vi "_UTIL_Run_TestVector File.vi"() -> ()   [LabVIEW 2024]
uses:
  Control Definitions/Def FullCfg.ctl
  Control Definitions/Def BenchCfg.ctl
  Control Definitions/Def PumpCtlRefs.ctl
  Control Definitions/Def Bench Status.ctl
  Control Definitions/Ded Spec RNG.ctl
  Control Definitions/Ded LUT_Status.ctl
  Control Definitions/Def Results2.ctl
panel:
  out "Time":dbl
  out "Point #":i32
  out "File Name":string
  out "Root path":path
  out "Results out":T1=[[{"Fill"=0.0, "Drain"=7.612782182151588, "Status"=5, "Resistor"=100.2}, {"Fill"=3.699999999999991, "Drain"=7.368700152811735, "Status"=9, "Resistor"=100.4}], [{"Fill"=7.519750916870415, "Drain"=7.144624847188264, "Status"=5, "Resistor"=199.3}, {"Fill"=7.323685024449877, "Drain"=6.908545507334963, "Status"=5, "Resistor"=199.4}], [{"Fill"=7.101610391198044, "Drain"=6.69747457212714, "Status"=5, "Resistor"=298.5}, {"Fill"=6.859529034229828, "Drain"=6.46039489608802, "Status"=5, "Resistor"=298.4}], [{"Fill"=6.616447341075794, "Drain"=6.23331858190709, "Status"=5, "Resistor"=397.6}, {"Fill"=6.4163801039119805, "Drain"=6.007242603911981, "Status"=5, "Resistor"=397.6}], [{"Fill"=6.176299419315403, "Drain"=5.775164608801956, "Status"=5, "Resistor"=497.4}, {"Fill"=5.938219407090465, "Drain"=5.544086949877751, "Status"=5, "Resistor"=497.2}], [{"Fill"=5.733150488997555, "Drain"=5.331015342298288, "Status"=5, "Resistor"=597.7}, {"Fill"=5.478064761613692, "Drain"=5.0889339853300735, "Status"=5, "Resistor"=597.0}], [{"Fill"=5.25498979217604, "Drain"=4.853854981662591, "Status"=5, "Resistor"=697.7}, {"Fill"=5.02791347799511, "Drain"=4.634781356968215, "Status"=5, "Resistor"=697.0}], [{"Fill"=4.795835482885085, "Drain"=4.415707732273838, "Status"=5, "Resistor"=797.9}, {"Fill"=4.572760513447433, "Drain"=0.0, "Status"=5, "Resistor"=797.2}], [{"Fill"=4.368691931540343, "Drain"=3.9545527506112466, "Status"=5, "Resistor"=897.6}, {"Fill"=4.125610238386308, "Drain"=4.172626039119804, "Status"=10, "Resistor"=856.6}], [{"Fill"=3.90853728606357, "Drain"=0.0, "Status"=5, "Resistor"=998.1}, {"Fill"=3.68246130806846, "Drain"=3.7114710574572127, "Status"=10, "Resistor"=897.1}], [{"Fill"=3.45638533007335, "Drain"=3.389362805623472, "Status"=10, "Resistor"=998.3}, {"Fill"=3.200299266503668, "Drain"=3.010235391198044, "Status"=10, "Resistor"=997.4}]] {"Resistor" format="%.1f"; "Drain" format="%.3f"; "Fill" format="%.3f"}
  in  "aSpec Out":T2[](array[typedef])
  out "Fill!Drain":bool=TRUE
  in  "Full Config":T4={"Bench Config"={"Name"="OLR001", {"Step Levels"=0.05, "Tolerance"=0.01, "Sample Rate"=0.05, "Resistor"=100.0, "M Level Cal"=1.0, "[B Level Cal"=0.0, "Max Fill Rate"=0.025, "Empty Inches"=8.6, "Full Inches"=2.0}}, "Test Value Table "=[[98.0, 102.0, 7.91, 8.01, 7.55, 7.65, 98.0, 102.0, 7.685, 7.785, 7.325, 7.425], [197.0, 203.0, 7.46, 7.56, 7.1, 7.2, 197.0, 203.0, 7.235, 7.335, 6.875, 6.975], [296.0, 304.0, 7.01, 7.11, 6.65, 6.75, 296.0, 304.0, 6.785, 6.885, 6.425, 6.525], [395.0, 405.0, 6.56, 6.66, 6.2, 6.3, 395.0, 405.0, 6.335, 6.435, 5.975, 6.075], [494.0, 506.0, 6.11, 6.21, 5.75, 5.85, 494.0, 506.0, 5.885, 5.985, 5.525, 5.625], [593.0, 607.0, 5.66, 5.76, 5.3, 5.4, 593.0, 607.0, 5.435, 5.535, 5.075, 5.175], [692.0, 708.0, 5.21, 5.31, 4.85, 4.95, 692.0, 708.0, 4.985, 5.085, 4.625, 4.725], [791.0, 809.0, 4.76, 4.86, 4.4, 4.5, 791.0, 809.0, 4.535, 4.635, 4.175, 4.275], [890.0, 910.0, 4.31, 4.41, 3.95, 4.05, 890.0, 910.0, 4.085, 4.185, 3.725, 3.825], [989.0, 1011.0, 3.86, 3.96, 3.5, 3.6, 989.0, 1011.0, 3.635, 3.735, 3.275, 3.375], [1088.0, 1112.0, 3.41, 3.51, 3.05, 3.15, 1088.0, 1112.0, 3.185, 3.285, 2.825, 2.925], [0.0, 0.0, 0.0, 0.0, 0.0, 0.0, 0.0, 0.0, 0.0, 0.0, 0.0, 0.0]], "Table Col Titles"=[["Aohm Lo", "Aohm Hi", "A Fill Lo", "A Fill Hi", "A Drain Lo", "A Drain Hi", "Bohm Lo", "Bohm Hi", "B Fill Lo", "B Fill Hi", "B Drain Lo", "B Drain Hi"]], "Pump CtlRef In"={"Fill "=refnum, "Drain"=refnum, "Level PV"=refnum, "Flow Rate%"=refnum, "Run Test"=refnum, "Sim"=refnum, "Jog"=refnum, "Level SP"=refnum}, "Bench Status"={"Pump Status"=refnum, "Instrumnet\n Status"=refnum}}
  out "Data":dbl[](array[numeric])=[679.25, 100.2, 100.3, 1.009, 8.61311836797066]
  out "DataQ Input":T8(graph)={"Ch A   Ohms"=100.2, " Ch B  Ohms"=100.3, "Level"=1.009}
  out "Level PV":dbl=8.61311836797066
  out "ChB":dbl=100.3
  out "ChA":dbl=100.2
  out "data decimal":dbl[][](array[numeric]) format="%.4f"
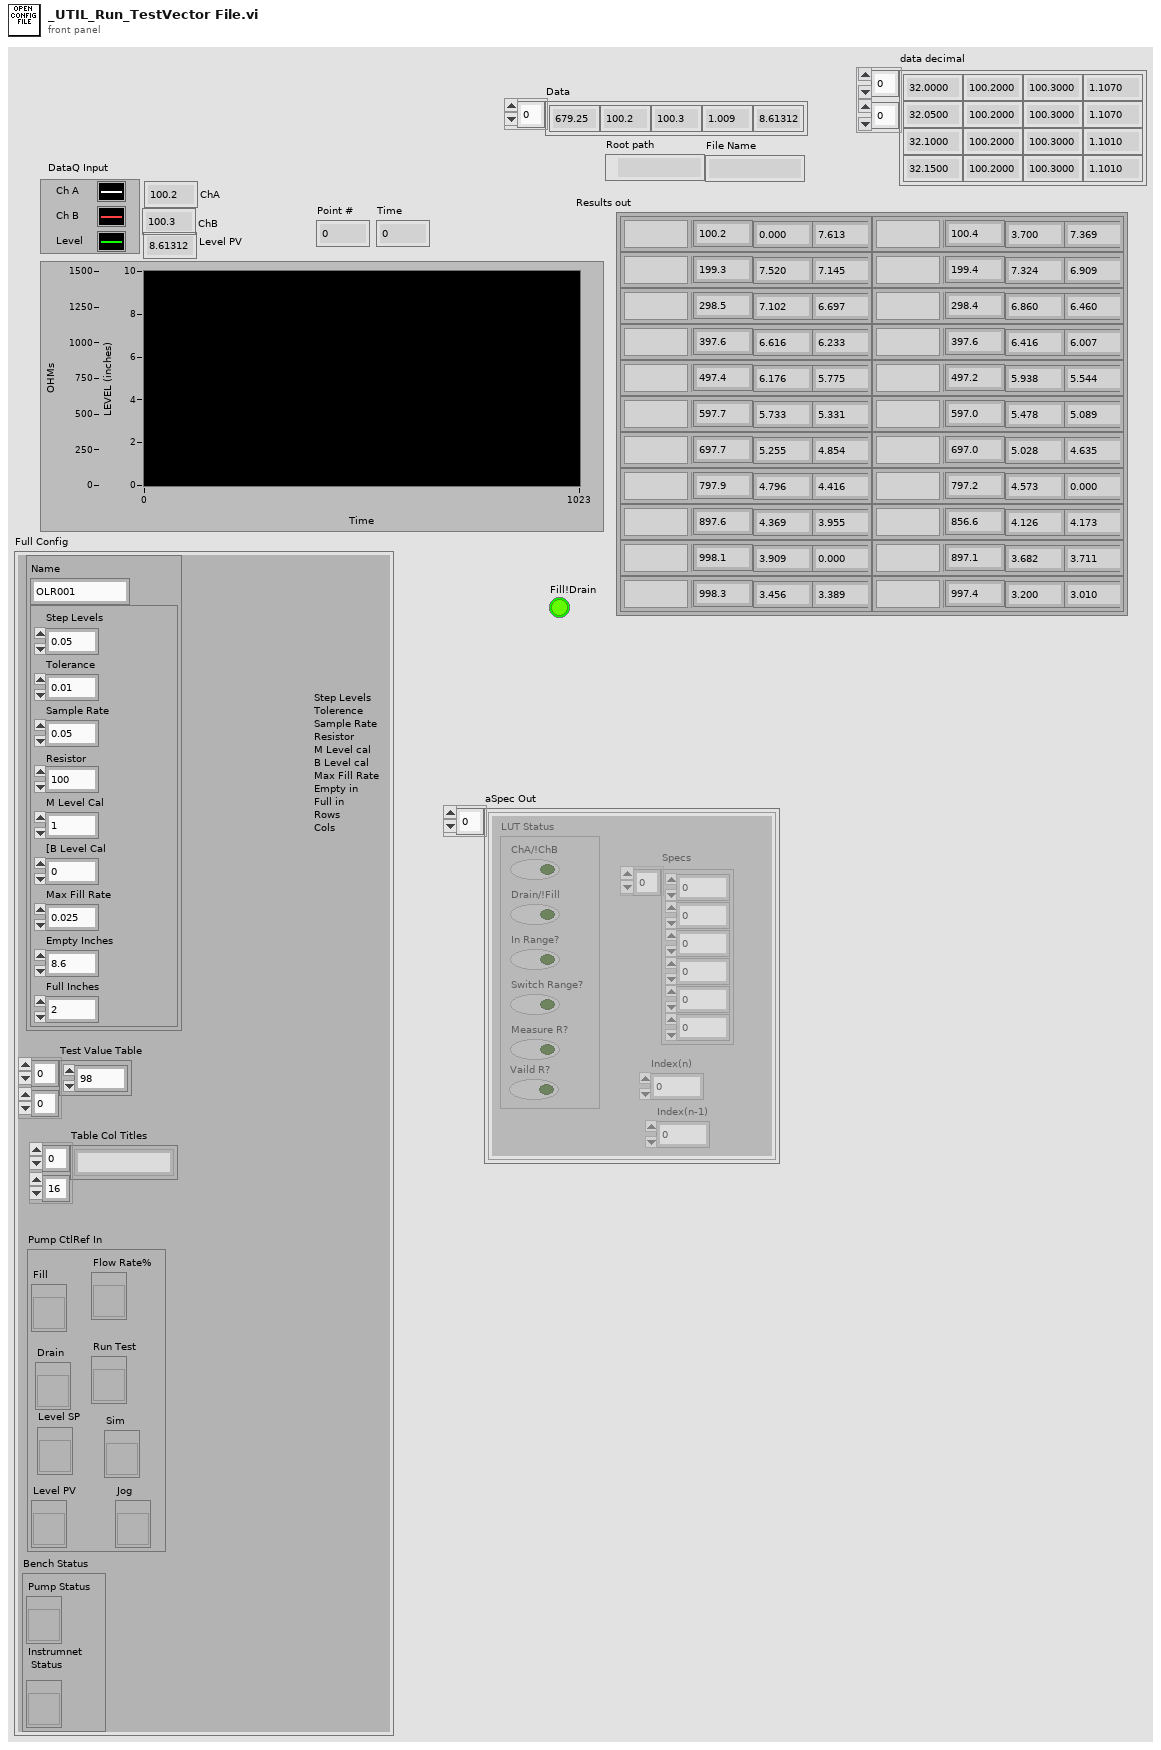
[diagram p1: front panel]
types:
  T1 = typedef "Def Results2.ctl" = cluster{"Fill":dbl, "Drain":dbl, "Status":i16, "Resistor":dbl}[][]
  T2 = typedef "Ded Spec RNG.ctl" = cluster{"Specs":dbl[], "Index(n)":i32, "LUT Status":T3, "Index(n-1)":i32}
  T3 = typedef "Ded LUT_Status.ctl" = cluster{"ChA/!ChB":bool, "Drain/!Fill":bool, "In Range?":bool, "Switch Range?":bool, "Measure R?":bool, "Vaild R?":bool}
  T4 = typedef "Def FullCfg.ctl" = cluster{"Bench Config":T5, "Test Value Table ":dbl[][], "Table Col Titles":string[][], "Pump CtlRef In":T6, "Bench Status":T7}
  T5 = typedef "Def BenchCfg.ctl" = cluster{"Name":string, cluster{"Step Levels":dbl, "Tolerance":dbl, "Sample Rate":dbl, "Resistor":dbl, "M Level Cal":dbl, "[B Level Cal":dbl, "Max Fill Rate":dbl, "Empty Inches":dbl, "Full Inches":dbl}}
  T6 = typedef "Def PumpCtlRefs.ctl" = cluster{"Fill ":refnum<vi>, "Drain":refnum<vi>, "Level PV":refnum<vi>, "Flow Rate%":refnum<vi>, "Run Test":refnum<vi>, "Sim":refnum<vi>, "Jog":refnum<vi>, "Level SP":refnum<vi>}
  T7 = typedef "Def Bench Status.ctl" = cluster{"Pump Status":refnum<vi>, "Instrumnet\n Status":refnum<vi>}
  T8 = cluster{"Ch A   Ohms":dbl, " Ch B  Ohms":dbl, "Level":dbl}
  T9 = cluster{"Ch A   Ohms":dbl, " Ch B  Ohms":dbl, "Level":dbl}[]
  T10 = cluster{"Resistor":dbl, "Fill":dbl, "Drain":dbl, "Status":i16}
  T11 = cluster{"Resistor":dbl, "Fill":dbl, "Drain":dbl, "Status":i16}[][]
  T12 = typedef "Def Measure.ctl" = cluster{"ChA R":dbl, "ChB R":dbl, "Level PV":dbl}
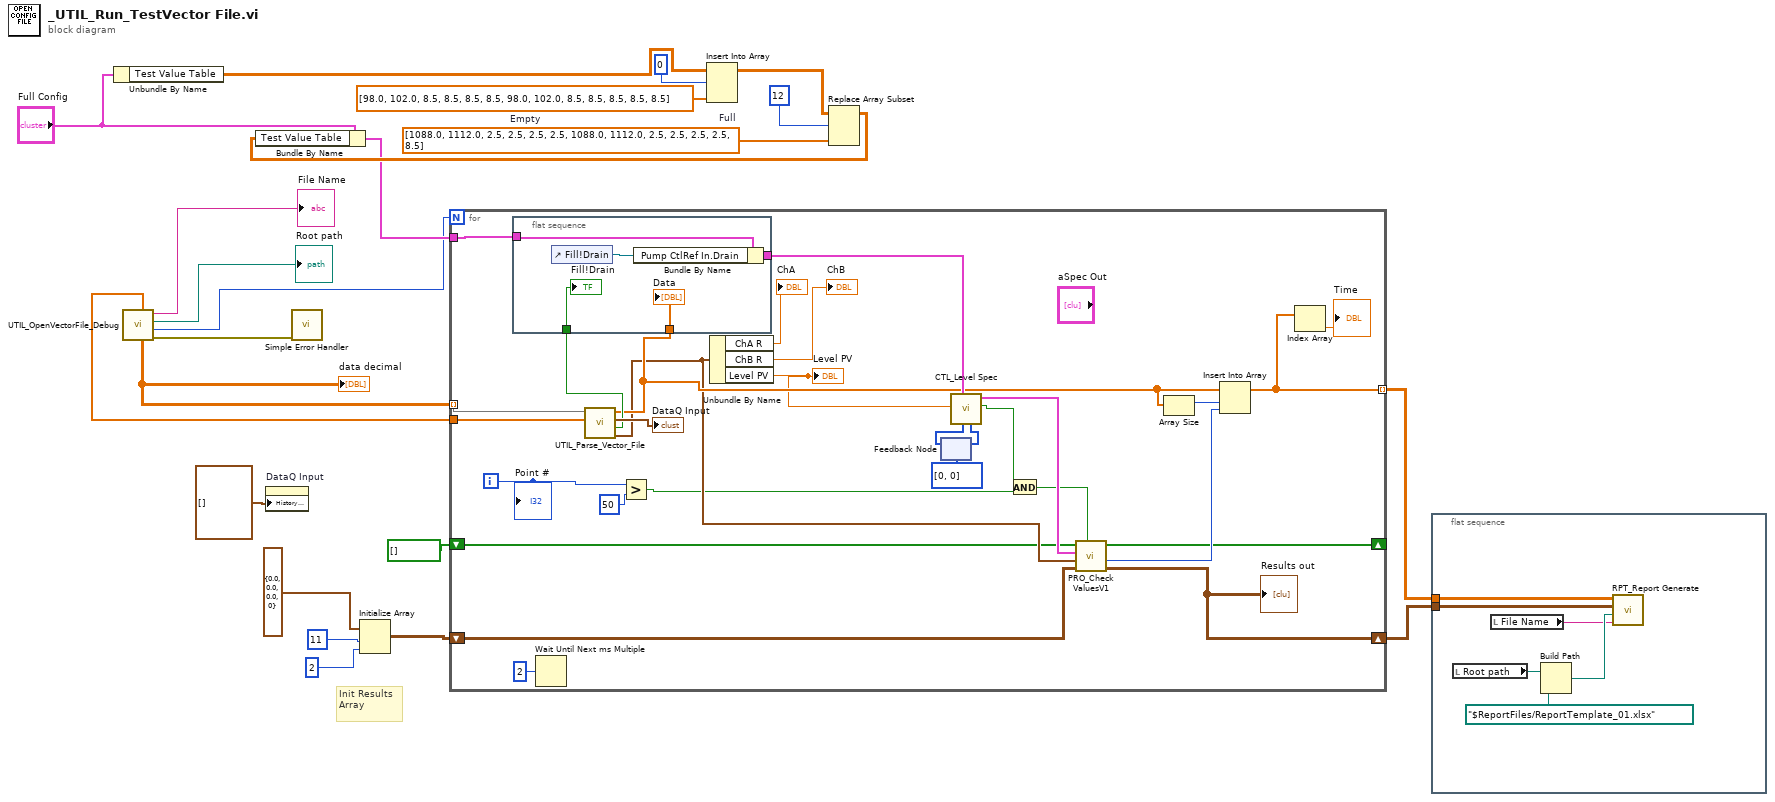
[diagram p0: block diagram]
diagram:
  w15 = dbl[] [1088.0, 1112.0, 2.5, 2.5, 2.5, 2.5, 1088.0, 1112.0, 2.5, 2.5, 2.5, 2.5, 8.5]  # Full
  w12 = dbl[] [98.0, 102.0, 8.5, 8.5, 8.5, 8.5, 98.0, 102.0, 8.5, 8.5, 8.5, 8.5, 8.5]  # Empty
  # "Init Results\nArray"
  n1 = Unbundle By Name("Full Config") -> ("Test Value Table"=w10:dbl[][])
  n2 = call "UTIL_OpenVectorFile_Debug.vi"() -> ("error out"=w1:errorcluster, "Numeric"=w2:i32, "path"=→"Root path":path, "before match"=→"File Name":string, "data 2"=w5:dbl[][], "data"=w6:dbl[])  [unwired: 6 in]
  "data decimal" <- w5
  n3 = property on="DataQ Input" class="WFChart (strict)"("History Data"=T9 []) -> ()  [unwired: 2 in, 2 out]
  n4 = call <vilib>:"Simple Error Handler.vi"("error in (no error)"=w1) -> ()  [unwired: 4 in, 5 out]
  n5 = Initialize Array(T10 {"Resistor"=0.0, "Fill"=0.0, "Drain"=0.0, "Status"=0} ("Cluster 2"), 11 ("dimension size"), 2 ("dimension size")) -> (w20:T11)
  n6 = Insert Into Array(array=w10, index (row)=0 ("disabled index (col)"), new element=w12) -> (w11:dbl[][])  [unwired: 1 in]
  n7 = Replace Array Subset(array=w11, new element=w15, index (row)=12 ("disabled index (col)")) -> (w9:dbl[][])  [unwired: 1 in]
  n8 = Bundle By Name(cluster="Full Config", "Test Value Table"=w9) -> (w8:T4)
  n9 = for {
    N: w2 -> [_]
    tunnel: w5 -> [w50] mode=indexing
    tunnel: w8 -> [w49]
    shift-right: [w44] -> w18
    shift-left: w20 -> [w43]
    tunnel: [w31] -> w19 mode=indexing
    tunnel: w6 -> [w39]
    shift-right: [w33] -> _
    shift-left: bool[] [] ("Switched In") -> [w34]
    i -> [w41]
    n10 = flat-sequence {
      tunnel: w49 -> [w57]
      tunnel: [w55] -> w46
      tunnel: w42 -> [w54]
      tunnel: w36 -> [w53]
      frame #0 {
        n11 = control-ref of="Fill!Drain"() -> (w56:refnum<vi>)
        n12 = Bundle By Name(cluster=w57, "Pump CtlRef In.Drain"=w56) -> (w55:T4)
        "Data" <- w53
        "Fill!Drain" <- w54
      }
    }
    n13 = Wait Until Next ms Multiple(millisecond multiple=u32 2) -> ()  [unwired: 1 out]
    n14 = call "UTIL_Parse_Vector_File.vi"("Cal Coef"=w39, "Data IN"=w50) -> ("Measure"=w35:T12, "Drain!Fill"=w42:bool, "Chart Data"=→"DataQ Input":cluster{dbl, dbl, dbl}, "Data Out"=w36:dbl[])  [unwired: 6 in]
    n15 = Greater?(x=w41, y=50) -> (0:w29:bool)
    n16 = Unbundle By Name(w35) -> ("ChA R"=→"ChA":dbl, "ChB R"=→"ChB":dbl, "Level PV"=w24:dbl)
    "Level PV" <- w24
    n17 = feedback #1(i32[] [0, 0] ("Index(n-1) In")) -> (w25:i32[])
    n18 = call "CTL_Level Spec.vi"("Index(n-1) In"=w25, "Full Config"=w46, "Level IN inches"=w24) -> ("Enable"=w27:bool, "aSpec Out"=w45:T2[], "Index(n-1) Out"=w26:i32[])  [unwired: 5 in, 1 out]
    n19 = feedback-in #1(w26) -> ()
    n20 = And(x=w27, y=w29) -> (x .and. y?=w28:bool)
    n21 = call "PRO_Check ValuesV1.vi"("Enable"=w28, "Results in"=w43, "Measure In"=w35, "aSpec In"=w45, "Switched In"=w34) -> ("Results out"=w44:T1, "Status Code"=w38:i32, "Switched Out"=w33:bool[])  [unwired: 3 in, 1 out]
    "Results out" <- w44
    n22 = Array Size(array=w36) -> (size(s)=w37:i32)
    n23 = Insert Into Array(array=w36, index=w37, new element=w38) -> (w31:dbl[])
    n24 = Index Array(array=w31) -> (element=→"Time":dbl)  [unwired: 1 in]
    "Point #" <- w41
  }
  n25 = flat-sequence {
    tunnel: w19 -> [w63]
    tunnel: w18 -> [w62]
    frame #0 {
      n26 = local read "Root path"() -> (w60:path)
      n27 = local read "File Name"() -> (w58:string)
      n28 = Build Path(base path=w60, name or relative path=path "$ReportFiles/ReportTemplate_01.xlsx") -> (appended path=w59:path)
      n29 = call "RPT_Report Generate.vi"("Report Name"=w58, "template"=w59, "Results"=w62, "Wave Data"=w63) -> ()  [unwired: 8 in]
    }
  }
